vi "Test Positive Definite.vi"   [LabVIEW 2017, in "NI_AALPro.lvlib"]
doc: "Tests whether <B>Input Matrix</B> is a complex-conjugate symmetric and positive definite matrix. The data type you wire to the <B>Input Matrix</B> input determines the polymorphic instance to use."
uses:
  <vilib>/Analysis/NI_AALPro.lvlib
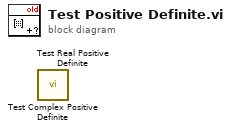
[diagram p0: block diagram]
diagram:
  n1 = call <vilib>:"Test Complex Positive Definite.vi"() -> ()  [unwired: 1 in, 2 out]
  n2 = call <vilib>:"Test Real Positive Definite.vi"() -> ()  [unwired: 1 in, 2 out]
